vi "TCPsendCommand.vi"(0 "DashboardServer in":refnum<class "Dashboard Server.lvclass">, 1 "command":string, 2 "data":string, 5 "error in (no error)":errorcluster) -> (14 "DashboardServer out":refnum<class "Dashboard Server.lvclass">, 15 "returnStatus":string, 16 "data":string, 19 "error out":errorcluster)   [LabVIEW 2016, in "Dashboard Server.lvclass"]
uses:
  Dashboard Server.lvclass
  <vilib>/Utility/error.llb/whitespace.ctl
  Dashboard Server.lvclass/Dashboard Server.ctl
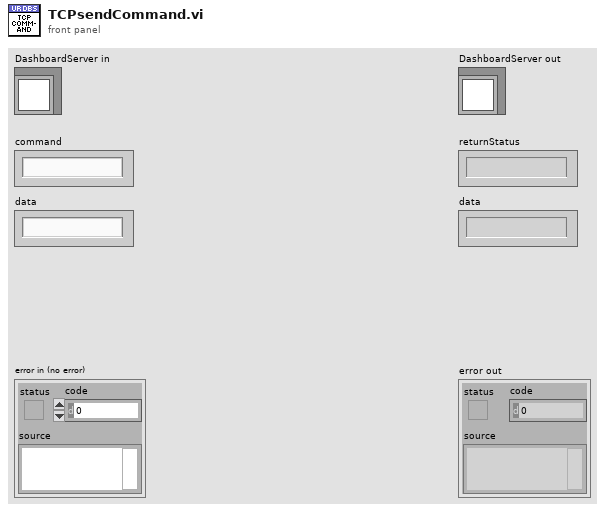
[diagram p1: front panel]
types:
  T1 = enum16{"Standard", "Buffered", "CRLF", "Immediate"}
  T2 = typedef "whitespace.ctl" = u16
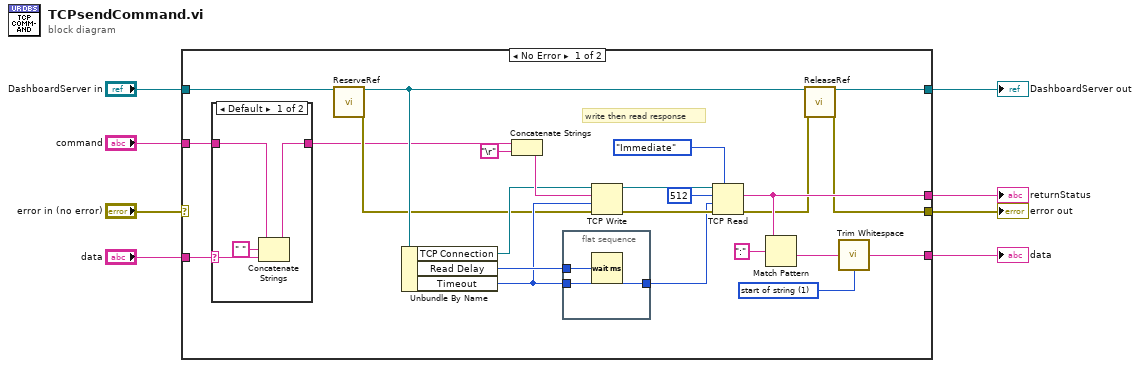
[diagram p0: block diagram]
diagram:
  n1 = case shown="No Error" "error in (no error)" {
    selector: "error in (no error)" -> [_ w41]
    tunnel: [w16 w41] -> w8
    tunnel: [w18 w40] -> w7
    tunnel: "DashboardServer in" -> [w20 w40]
    tunnel: "command" -> [w10 _]
    tunnel: [w12 _] -> w5
    tunnel: [w21 _] -> w6
    tunnel: "data" -> [w11 _]
    frame No Error {
      w13 = T2 1 items=["both", "start of string", "end of string"] ("location (both)")
      # "write then read response"
      n2 = case shown="Default" w11 {
        selector: w11 -> [w35 _]
        tunnel: w10 -> [w36 w37]
        tunnel: [w34 w37] -> w9
        frame Default {
          n3 = Concatenate Strings(w36, " " ("string"), w35) -> (w34:string)
        }
        frame "" {
        }
      }
      n4 = call "ReserveRef.vi"("DashboardServer in"=w20) -> ("DashboardServer out"=w19:refnum<class "Dashboard Server.lvclass">, "error out"=w15:errorcluster)  [unwired: 17 in]
      n5 = Unbundle By Name(w19) -> ("TCP Connection"=w27:refnum<k5>, "Read Delay"=w25:u32, "Timeout"=w24:i32)
      n6 = Concatenate Strings(w9, "\r") -> (w29:string)
      n7 = flat-sequence {
        tunnel: w25 -> [w39]
        tunnel: w24 -> [w38]
        tunnel: [w38] -> w22
        frame #0 {
          n8 = Wait (ms)(milliseconds to wait=w39) -> ()  [unwired: 1 out]
        }
      }
      n9 = TCP Write(connection ID=w27, data in=w29, error in (no error)=w15, 9:w24) -> (connection ID out=w26:refnum<k5>, error out=w23:errorcluster)  [unwired: 1 out]
      n10 = TCP Read(connection ID=w26, bytes to read=512, error in (no error)=w23, 7:T1."Immediate" ("mode (standard)"), 9:w22) -> (data out=w21:string, error out=w17:errorcluster)  [unwired: 1 out]
      n11 = Match Pattern(string=w21, regular expression=":") -> (after substring=w14:string)  [unwired: 1 in, 3 out]
      n12 = call "ReleaseRef.vi"("DashboardServer in"=w19, "error in (no error)"=w17) -> ("DashboardServer out"=w18:refnum<class "Dashboard Server.lvclass">, "error out"=w16:errorcluster)  [unwired: 16 in]
      n13 = call <vilib>:"Trim Whitespace.vi"("string"=w14, "location (both)"=w13) -> ("trimmed string"=w12:string)
    }
    frame Error {
    }
  }
  "error out" <- w8
  "DashboardServer out" <- w7
  "returnStatus" <- w6
  "data" <- w5
